vi "Read Stream Data File.vi"() -> ()   [LabVIEW 2020]
panel:
  out "Waveform Graph":dbl[](graph)
  in  "File Path":path
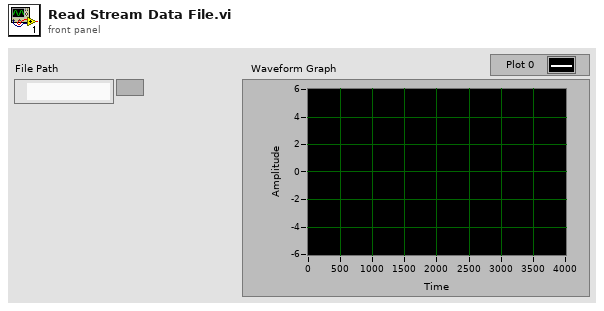
[diagram p1: front panel]
types:
  T1 = enum16{"open", "replace", "create", "open or create", "replace or create", "replace or create with confirmation"}
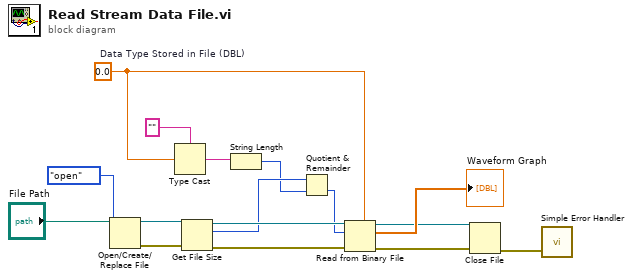
[diagram p0: block diagram]
diagram:
  w10 = 0.0  # Data Type Stored in File (DBL)
  n1 = Open/Create/Replace File(file path (use dialog)="File Path", operation (0:open)=T1."open") -> (refnum out=w14:refnum<file>, error out=w12:errorcluster)  [unwired: 4 in, 1 out]
  n2 = Type Cast(type="", x=w10) -> (*(type *) &x=w8:string)
  n3 = Get File Size(file=w14, error in=w12) -> (refnum out=w13:refnum<file>, size (in bytes)=w7:i64, 0:w11:errorcluster)
  n4 = String Length(string=w8) -> (length=w6:i32)
  n5 = Quotient & Remainder(x=w7, y=w6) -> (floor(x/y)=w5:i64)  [unwired: 1 out]
  n6 = Read from Binary File(5:w10, 8:w11, 10:w5, 11:w13) -> (0:w2:errorcluster, 2:→"Waveform Graph":dbl[], 3:w3:refnum<file>)  [unwired: 2 in, 1 out]
  n7 = Close File(refnum=w3, error in=w2) -> (error out=w1:errorcluster)  [unwired: 1 out]
  n8 = call <vilib>:"Simple Error Handler.vi"("error in (no error)"=w1) -> ()  [unwired: 4 in, 5 out]
